vi "CSTK_Icon_Creator_Insert_TitleText.vi"(5 "字体":enum16{"Small Fonts", "6px2bus"}(ring), 6 "水平偏移":i8, 7 "LOGO":string, 8 "error in (no error)":errorcluster, 9 "字符":string, 10 "字体颜色":u32, 11 "图片输入":picture) -> (0 "error out":errorcluster, 3 "图片输出":picture)   [LabVIEW 2015, in "CSTK_Icon Creator.lvlib"]
uses:
  CSTK_Icon Creator.lvlib
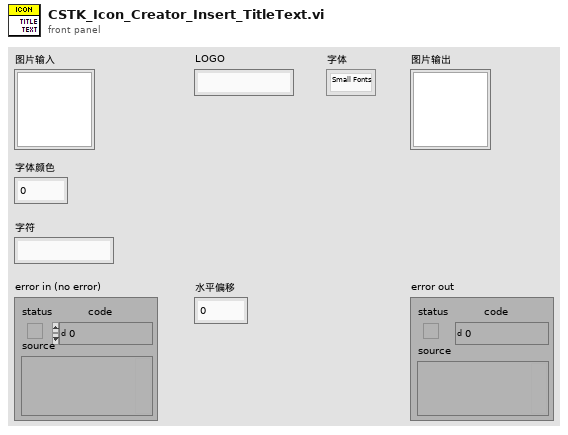
[diagram p1: front panel]
types:
  T1 = enum16{"User-specified Font", "Application Font", "System Font", "Dialog Font"}
  T2 = cluster{"left":i16, "top":i16, "right":i16, "bottom":i16}
  T3 = cluster{"Font Name:":string, "Size":i16, "Strikeout?":bool, "Italic?":bool, "Underline?":bool, "Outline?":bool, "Shadow?":bool, "Bold?":bool}
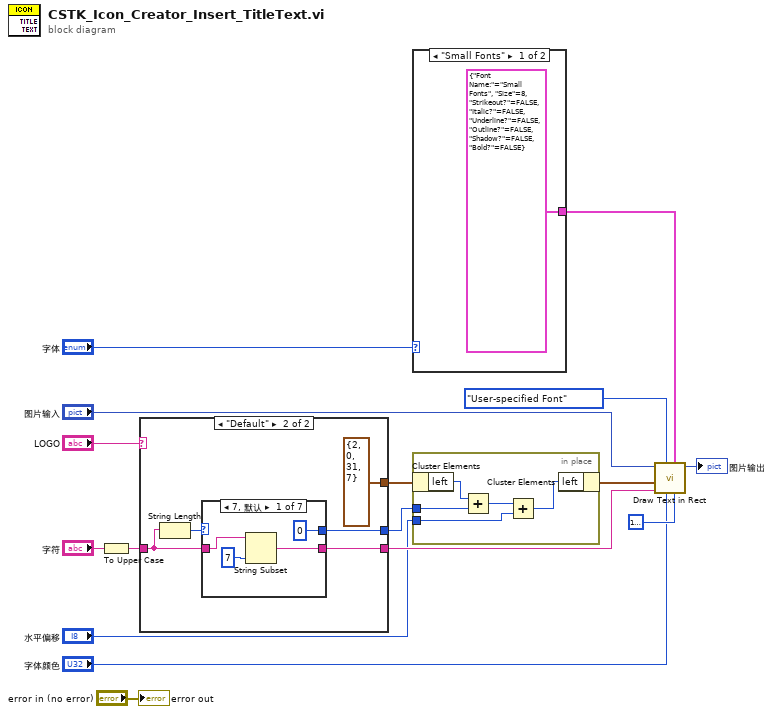
[diagram p0: block diagram]
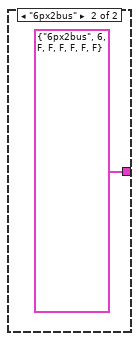
[diagram p2: hidden frame]
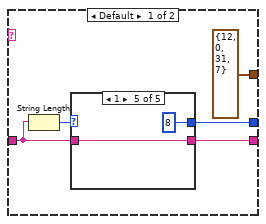
[diagram p3: hidden frame]
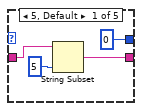
[diagram p4: hidden frame]
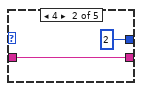
[diagram p5: hidden frame]
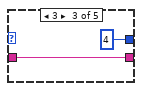
[diagram p6: hidden frame]
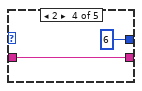
[diagram p7: hidden frame]
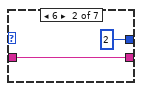
[diagram p8: hidden frame]
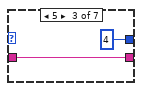
[diagram p9: hidden frame]
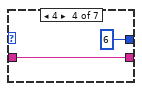
[diagram p10: hidden frame]
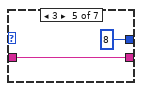
[diagram p11: hidden frame]
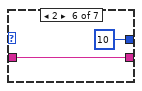
[diagram p12: hidden frame]
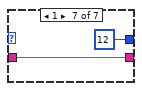
[diagram p13: hidden frame]
diagram:
  n1 = To Upper Case(1:"字符") -> (0:w1:string)
  n2 = case shown="\"Default\"" "LOGO" {
    tunnel: [T2 {"left"=12, "top"=0, "right"=31, "bottom"=7} ("rect") T2 {"left"=2, "top"=0, "right"=31, "bottom"=7} ("rect")] -> w14
    tunnel: [w20 w37] -> w13
    tunnel: w1 -> [w17 w34]
    tunnel: [w18 w35] -> w4
    frame Default {
      n3 = String Length(string=w17) -> (length=w19:i32)
      n4 = case shown="1" w19 {
        tunnel: [i16 0 i16 2 i16 4 i16 6 i16 8] -> w20
        tunnel: [w23 w26 w28 w30 w32] -> w18
        tunnel: w17 -> [w24 w26 w28 w30 w32]
        frame 5, Default {
          n5 = String Subset(string=w24, length (rest)=5 ("长度（剩余）")) -> (substring=w23:string)  [unwired: 1 in]
        }
        frame 4 {
        }
        frame 3 {
        }
        frame 2 {
        }
        frame 1 {
        }
      }
    }
    frame "Default" {
      n6 = String Length(string=w34) -> (length=w36:i32)
      n7 = case shown="7, 默认" w36 {
        tunnel: [i16 0 i16 2 i16 4 i16 6 i16 8 i16 10 i16 12] -> w37
        tunnel: [w40 w43 w45 w47 w49 w51 w53] -> w35
        tunnel: w34 -> [w41 w43 w45 w47 w49 w51 w53]
        frame 7, Default {
          n8 = String Subset(string=w41, length (rest)=7 ("长度（剩余）")) -> (substring=w40:string)  [unwired: 1 in]
        }
        frame 6 {
        }
        frame 5 {
        }
        frame 4 {
        }
        frame 3 {
        }
        frame 2 {
        }
        frame 1 {
        }
      }
    }
  }
  n9 = case shown="\"Small Fonts\"" "字体" {
    tunnel: [T3 {"Font Name:"="Small Fonts", "Size"=8, "Strikeout?"=FALSE, "Italic?"=FALSE, "Underline?"=FALSE, "Outline?"=FALSE, "Shadow?"=FALSE, "Bold?"=FALSE} ("[user-specified font]") T3 {"Font Name:"="6px2bus", "Size"=6, "Strikeout?"=FALSE, "Italic?"=FALSE, "Underline?"=FALSE, "Outline?"=FALSE, "Shadow?"=FALSE, "Bold?"=FALSE} ("[user-specified font]")] -> w8
    frame "Small Fonts" {
    }
    frame "6px2bus" {
    }
  }
  n10 = in-place {
    in-place-border: w13 -> [w60]
    in-place-border: "水平偏移" -> [w57]
    n11 = in-place-cluster #1(w14) -> ("left"=w61:i16)
    n12 = Add(x=w61, y=w60) -> (x+y=w59:i16)
    n13 = Add(x=w59, y=w57) -> (x+y=w58:i16)
    n14 = in-place-cluster #1("left"=w58) -> (w15:T2)
  }
  n15 = call <vilib>:"Draw Text in Rect.vi"("BG color(transparent)"=u32 16777216, "[user-specified font]"=w8, "text color(black)"="字体颜色", "desired font(Application)"=T1."User-specified Font", "text"=w4, "rect"=w15, "picture"="图片输入") -> ("new picture"=→"图片输出":picture)  [unwired: 4 in]
  "error out" <- "error in (no error)"
